vi "Triple coincidence.vi"() -> ()   [LabVIEW 2012]
panel:
  in  "Save file":bool
  in  "Comment":string
  out "Start time":u32
  out "XY Graph":cluster{"Y":dbl[], "Y":dbl[]}[](graph)
  in  "Histogram on/off":bool
  in  "Set window1":bool
  in  "Channel3 Pulse Front":string(combo)
  in  "Channel2 Pulse Front":string(combo)
  out "Waveform Graph 4":cluster{i16, dbl, "Array":i64[]}(graph) caption="Ch1-Ch3"
  out "Waveform Graph 3":cluster{i16, dbl, "Array":i64[]}(graph) caption="Ch1-Ch2"
  out "Waveform Graph 2":cluster{i16, dbl, "Array":i64[]}(graph) caption="Waveform Graph2"
  in  "Window Offset 2 (ns)":i32
  in  "Window Length 2 (ns)":i32
  in  "Window Offset 1 (ns)":i32
  in  "Window Length 1 (ns)":i32
  out "Waveform Graph 1":cluster{i16, dbl, "Array":i64[]}(graph) caption="Waveform Graph"
  out "Single Count Channel3":i64 format="%_3p"
  out "Single Count Channel2":i64 format="%_3p"
  out "Single Count Channel1":i64 format="%_3p"
  out "Exposition time (ms)":i64
  out "Measurement index":i64
  out "Start OK":bool
  in  "Exit":bool
  in  "Channel3 Threshold Voltage (mV)":i32
  in  "Channel2 Threshold Voltage (mV)":i32
  in  "Channel1 Pulse Front":string(combo)
  in  "Channel1 Threshold Voltage (mV)":i32 min=0 max=5000 step=10
  in  "Exposition Time (ms)":i64
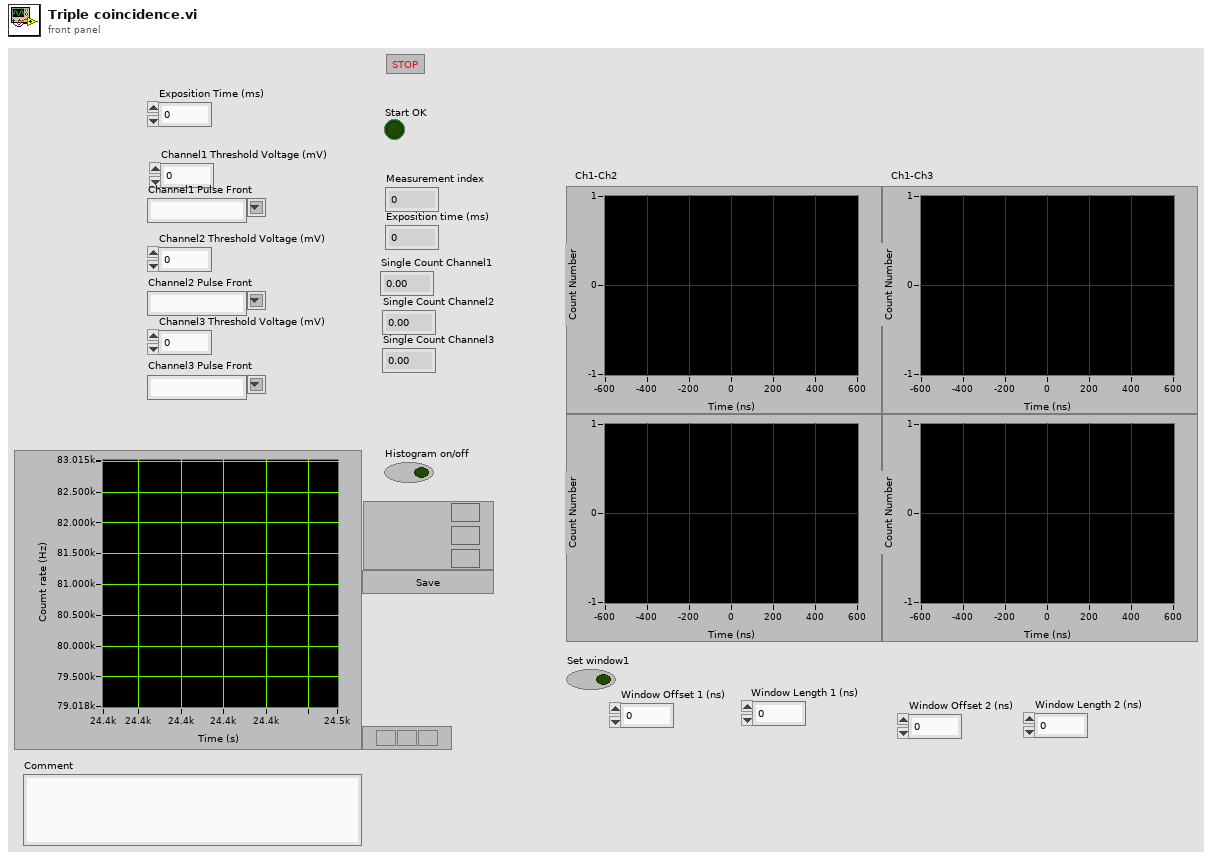
[diagram p1: front panel]
types:
  T1 = cluster{"Channel1":bool, "Channel2":bool, "Channel3":bool, "Channel4":bool}
  T2 = cluster{"Stop Channel":string, "Start Channel":string}
  T3 = cluster{"[0]":i64, "Channel1 Threshold Voltage (mV)":i32, "Channel1 Pulse Front":string, "Channel2 Threshold Voltage (mV)":i32, "Channel2 Pulse Front":string, "Channel3 Threshold Voltage (mV)":i32, "Channel3 Pulse Front ":string, "Channel4 Threshold Voltage (mV)":i32, "Channel4 Pulse Front ":string, "Single Count Enable":cluster{"Channel1":bool, "Channel2":bool, "Channel3":bool, "Channel4":bool}, "Single Count Max":i32, "Sum Count Enable":cluster{"Channel1":bool, "Channel2":bool, "Channel3":bool, "Channel4":bool}, "Sum Count Max":i32, "Start-Stop1 Multyplex":cluster{"Stop Channel":string, "Start Channel":string}, "Stop Delay 1 (ns)":i16, "Window Length 1 (ns)":i32, "Window Offset 1 (ns) ":i32, "Conditional Correlation 1":string, "Histogram Bin 1":string, "Histogram Start 1 (ns) ":i32, "Start-Stop2 Multyplex ":cluster{"Stop Channel":string, "Start Channel":string}, "Stop Delay 2 (ns)":i16, "Window Length 2 (ns) ":i32, "Window Offset 2 (ns) ":i32, "Conditional Correlation 2":string, "Histogram Bin 2":string, "Histogram Start 2 (ns)  ":i32, "Start-Stop3 Multyplex":cluster{"Stop Channel":string, "Start Channel":string}, "Stop Delay 3 (ns)":i16, "Window Length 3 (ns) ":i32, "Window Offset 3 (ns) ":i32, "Conditional Correlation 3":string, "Histogram Bin 3":string, "Histogram Start 3 (ns) ":i32, "Start-Stop4 Multyplex":cluster{"Stop Channel":string, "Start Channel":string}, "Stop Delay 4 (ns)":i16, "Window Length 4 (ns)  ":i32, "Window Offset 4 (ns) ":i32, "Conditional Correlation 4":string, "Histogram Bin 4":string, "Histogram Start 4 (ns)  ":i32, "Coincidence Count Enable":cluster{"Start-Stop1":bool, "Start-Stop2":bool, "Start-Stop3":bool, "Start-Stop4":bool}, "Coincidence Count Max":i32, "Coincidence Sum Enable":cluster{"Start-Stop1":bool, "Start-Stop2":bool, "Start-Stop3":bool, "Start-Stop4":bool}, "Coincidence Sum Max":i32, "Output Channel Enable":cluster{"Channel1":bool, "Channel2":bool, "Channel3":bool, "Channel4":bool}, "Output Channel Inversion":cluster{"Channel1":bool, "Channel2":bool, "Channel3":bool, "Channel4":bool, "Output":bool}}
  T4 = cluster{"Going":bool, "Iinterrupted":bool, "Timer stop":bool, "Single count stop Ch1":bool, "Single count stop Ch2":bool, "Single count stop Ch3":bool, "Single count stop Ch4":bool, "Sum count stop":bool, "Coincidence count stop SS1":bool, "Coincidence count stop SS2":bool, "Coincidence count stop SS3":bool, "Coincidence count stop SS4":bool, "Coincidence sum count stop":bool, "Reserved":bool, "Correlator is not initialised":bool, "Internal error":bool}
  T5 = cluster{"Measurement index":i64, "Exposition time (ms)":i64, "Single Count Channel1":i64, "Single Count Channel2":i64, "Single Count Channel3":i64, "Single Count Channel4":i64, "Sum Single Count":i64, "Coincidence Count SS1":i64, "Coincidence Count SS2":i64, "Coincidence Count SS4":i64, "Coincidence Count SS5":i64, "Sum Coincidence Count":i64}
  T6 = typedef "LVCursorListTypeDef.ctl" = cluster{"Name":string, "Color":u32, "Style":u8, "Point Style":u8, "Name Visible":bool, "Allow Drag":bool, "Cursor Mode":u32, "Plot":i32, "Index":i32, "Position":cluster{"X":dbl, "Y":dbl}, "X Scale":u32, "Y Scale":u32, "Watch Plots":i32[], "Watch All Plots":bool, "Plot Area":i32, "Label Offset":cluster{"X":dbl, "Y":dbl}}[]
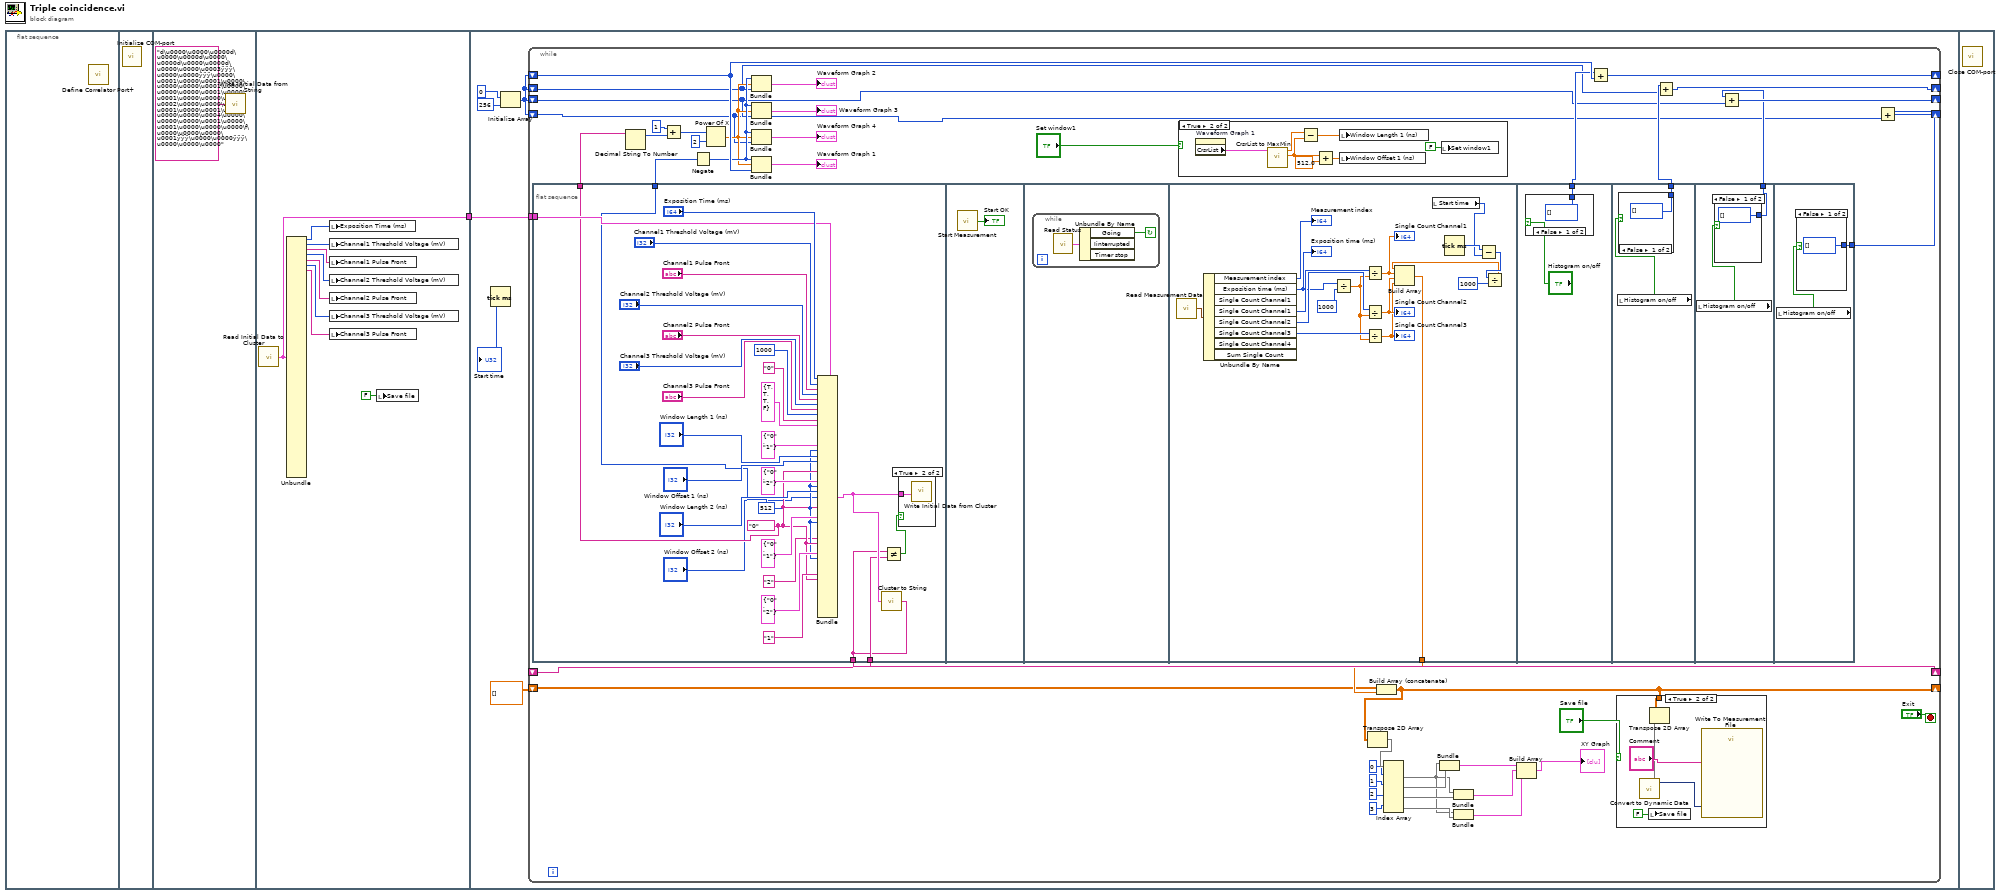
[diagram p0: block diagram]
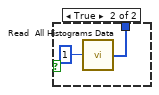
[diagram p5: hidden frame]
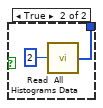
[diagram p6: hidden frame]
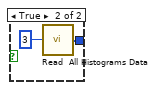
[diagram p7: hidden frame]
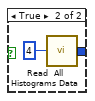
[diagram p8: hidden frame]
diagram:
  n1 = flat-sequence {
    tunnel: [w11] -> w1
    tunnel: w1 -> [w17]
    frame #0 {
      n2 = call "Define Correlator Port+.vi"() -> ()  [unwired: 3 in]
    }
    frame #1 {
      n3 = call "Initialize COM-port.vi"() -> ()  [unwired: 4 in]
    }
    frame #2 {
      n4 = call "Write Initial Data from String.vi"("Data"="d\u0000\u0000\u0000d\u0000\u0000d\u0000\u0000d\u0000\u0000d\u0000\u0000\u0003ÿÿÿ\u0000\u0000ÿÿÿ\u0000\u0001\u0000\u0001\u0000\u0000\u0000\u0001\u0000\u0000\u0000\u0001\u0000\u0001\u0000\u0000\u0000\u0002\u0000\u0000\u0000\u0001\u0000\u0001\u0000\u0000\u0000\u0004\u0000\u0000\u0000\u0001\u0000\u0001\u0000\u0000\u0000\f\u0000\u0000\u0000\u0001ÿÿÿ\u0000\u0000ÿÿÿ\u0000\u0000\u0000") -> ()  [unwired: 1 out]
    }
    frame #3 {
      n5 = call "Read Initial Data to Cluster.vi"() -> ("Correlator Initial Data 2"=w11:T3)  [unwired: 2 in]
      n6 = Unbundle(w11) -> ("[0]"=w10:i64, "Channel1 Threshold Voltage (mV)"=w9:i32, "Channel1 Pulse Front"=w8:string, "Channel2 Threshold Voltage (mV)"=w7:i32, "Channel2 Pulse Front"=w5:string, "Channel3 Threshold Voltage (mV)"=w6:i32, "Channel3 Pulse Front"=w4:string)  [unwired: 40 out]
      n7 = local write "Exposition Time (ms)"(w10) -> ()
      n8 = local write "Channel1 Threshold Voltage (mV)"(w9) -> ()
      n9 = local write "Channel1 Pulse Front"(w8) -> ()
      n10 = local write "Channel2 Threshold Voltage (mV)"(w7) -> ()
      n11 = local write "Channel2 Pulse Front"(w5) -> ()
      n12 = local write "Channel3 Threshold Voltage (mV)"(w6) -> ()
      n13 = local write "Channel3 Pulse Front"(w4) -> ()
      n14 = local write "Save file"(FALSE ("Save file")) -> ()
    }
    frame #4 {
      n15 = Tick Count (ms)() -> (millisecond timer value=→"Start time":u32)
      n16 = Initialize Array(i64 0 ("Value"), 256 ("dimension size")) -> (w14:i64[])
      n17 = while {
        tunnel: w17 -> [w62]
        shift-right: [w61] -> _
        shift-left: w14 -> [w53]
        shift-right: [w46] -> _
        shift-left: w14 -> [w40]
        shift-right: [w45] -> _
        shift-left: w14 -> [w39]
        shift-right: [w41] -> _
        shift-left: w14 -> [w38]
        shift-right: [w37] -> _
        shift-left: _ -> [w36]
        shift-right: [w19] -> _
        shift-left: dbl[][] [] -> [w33]
        stop <- "Exit" stop-if-true
        n18 = flat-sequence {
          tunnel: w62 -> [w97]
          tunnel: [w82] -> w59
          tunnel: [w86] -> w58
          tunnel: [w77] -> w37
          tunnel: w36 -> [w78]
          tunnel: [w112] -> w34
          tunnel: [w125] -> w52
          tunnel: [w130] -> w44
          tunnel: [w135] -> w43
          tunnel: [w140] -> w42
          frame #0 {
            w86 = "0" ("Histogram Bin")
            w82 = i16 512 ("Stop Delay1  (ns)")
            n19 = Bundle(cluster=w97, "[0]"="Exposition Time (ms)", "Channel1 Threshold Voltage (mV)"="Channel1 Threshold Voltage (mV)", "Channel1 Pulse Front"="Channel1 Pulse Front", "Channel2 Threshold Voltage (mV)"="Channel2 Threshold Voltage (mV)", "Channel2 Pulse Front"="Channel2 Pulse Front", "Channel3 Threshold Voltage (mV)"="Channel3 Threshold Voltage (mV)", "Channel3 Pulse Front"="Channel3 Pulse Front", "Channel4 Threshold Voltage (mV)"=1000, "Channel4 Pulse Front"="0", "Single Count Enable"=T1 {"Channel1"=TRUE, "Channel2"=TRUE, "Channel3"=TRUE, "Channel4"=FALSE}, "Start-Stop1 Multyplex"=T2 {"Stop Channel"="0", "Start Channel"="1"}, "Stop Delay 1 (ns)"=w82, "Window Length 1 (ns)"="Window Length 1 (ns)", "Window Offset 1 (ns)"="Window Offset 1 (ns)", "Histogram Bin 1"=w86, "Start-Stop2 Multyplex"=T2 {"Stop Channel"="0", "Start Channel"="2"}, "Stop Delay 2 (ns)"=w82, "Window Length 2 (ns)"="Window Length 2 (ns)", "Window Offset 2 (ns)"="Window Offset 2 (ns)", "Histogram Bin 2"=w86, "Start-Stop3 Multyplex"=T2 {"Stop Channel"="0", "Start Channel"="1"}, "Stop Delay 3 (ns)"=w82, "Conditional Correlation 3"="2", "Histogram Bin 3"=w86, "Start-Stop4 Multyplex"=T2 {"Stop Channel"="0", "Start Channel"="2"}, "Stop Delay 4 (ns)"=w82, "Conditional Correlation 4"="1", "Histogram Bin 4"=w86) -> (w79:T3)  [unwired: 19 in]
            n20 = call "Cluster to String.vi"("Correlator Initial Data"=w79) -> ("string"=w77:string)
            n21 = Not Equal?(x=w77, y=w78) -> (x != y?=w76:bool)
            n22 = case shown="True" w76 {
              tunnel: w79 -> [_ w103]
              frame False {
              }
              frame True {
                n23 = call "Write Initial Data from Cluster.vi"("Correlator Initial Data"=w103) -> ()  [unwired: 2 in, 1 out]
              }
            }
          }
          frame #1 {
            n24 = call "Start Measurement.vi"() -> ("Start OK"=→"Start OK":bool)  [unwired: 2 in]
          }
          frame #2 {
            n25 = while {
              stop <- w105 continue-if-true
              n26 = call "Read Status.vi"() -> ("Status Data"=w106:T4)  [unwired: 2 in]
              n27 = Unbundle By Name(w106) -> ("Going"=w105:bool)  [unwired: 2 out]
            }
          }
          frame #3 {
            n28 = call "Read Measurement Data.vi"() -> ("Measurement Data"=w122:T5)  [unwired: 3 in]
            n29 = Unbundle By Name(w122) -> ("Measurement index"=→"Measurement index":i64, "Exposition time (ms)"=w114:i64, "Single Count Channel1"=w121:i64, "Single Count Channel2"=w118:i64, "Single Count Channel3"=w117:i64)  [unwired: 3 out]
            "Exposition time (ms)" <- w114
            n30 = Divide(x=w114, y=i64 1000) -> (x/y=w115:dbl)
            n31 = Divide(x=w121, y=w115) -> (x/y=w120:dbl)
            "Single Count Channel1" <- w120
            n32 = Divide(x=w118, y=w115) -> (x/y=w119:dbl)
            "Single Count Channel2" <- w119
            n33 = Divide(x=w117, y=w115) -> (x/y=w116:dbl)
            "Single Count Channel3" <- w116
            n34 = local read "Start time"() -> (w110:u32)
            n35 = Tick Count (ms)() -> (millisecond timer value=w111:u32)
            n36 = Subtract(x=w111, y=w110) -> (x-y=w109:u32)
            n37 = Divide(x=w109, y=u32 1000) -> (x/y=w107:dbl)
            n38 = Build Array(w107, w120, w119, w116) -> (w112:dbl[])
          }
          frame #4 {
            n39 = case shown="False" "Histogram on/off" {
              tunnel: [i64[] [] ("Array") w127] -> w125
              frame False {
              }
              frame True {
                n40 = call "Read  All Histograms Data.vi"("Start-Stop#"=i8 1) -> ("Array"=w127:i64[])
              }
            }
          }
          frame #5 {
            n41 = local read "Histogram on/off"() -> (w129:bool)
            n42 = case shown="False" w129 {
              tunnel: [i64[] [] ("Array") w132] -> w130
              frame False {
              }
              frame True {
                n43 = call "Read  All Histograms Data.vi"("Start-Stop#"=i8 2) -> ("Array"=w132:i64[])
              }
            }
          }
          frame #6 {
            n44 = local read "Histogram on/off"() -> (w134:bool)
            n45 = case shown="False" w134 {
              tunnel: [i64[] [] ("Array") w137] -> w135
              frame False {
              }
              frame True {
                n46 = call "Read  All Histograms Data.vi"("Start-Stop#"=i8 3) -> ("Array"=w137:i64[])
              }
            }
          }
          frame #7 {
            n47 = local read "Histogram on/off"() -> (w139:bool)
            n48 = case shown="False" w139 {
              tunnel: [i64[] [] ("Array") w142] -> w140
              frame False {
              }
              frame True {
                n49 = call "Read  All Histograms Data.vi"("Start-Stop#"=i8 4) -> ("Array"=w142:i64[])
              }
            }
          }
        }
        n50 = Decimal String To Number(string=w58) -> (offset past number=w57:i32)  [unwired: 2 in, 1 out]
        n51 = Add(x=1, y=w57) -> (x+y=w54:i32)
        n52 = Negate(x=w59) -> (-x=w48:i16)
        n53 = Power Of X(1:i8 2 ("x"), 2:w54) -> (0:w47:dbl)
        n54 = Bundle(w48, w47, w40) -> (→"Waveform Graph 2":cluster{i16, dbl, i64[]})  [unwired: 1 in]
        n55 = Bundle(w48, w47, w39) -> (→"Waveform Graph 3":cluster{i16, dbl, i64[]})  [unwired: 1 in]
        n56 = Bundle(w48, w47, w38) -> (→"Waveform Graph 4":cluster{i16, dbl, i64[]})  [unwired: 1 in]
        n57 = Bundle(w48, w47, w53) -> (→"Waveform Graph 1":cluster{i16, dbl, i64[]})  [unwired: 1 in]
        n58 = case shown="True" "Set window1" {
          frame False {
          }
          frame True {
            n59 = property on="Waveform Graph 1" class="WFGraph (strict)"() -> ("CrsrList"=w75:T6)  [unwired: 2 in, 2 out]
            n60 = call "CrsrList to MaxMin.vi"("CrsrList"=w75) -> ("Min"=w73:dbl, "Max"=w74:dbl)  [unwired: 9 in]
            n61 = Subtract(x=w74, y=w73) -> (x-y=w71:dbl)
            n62 = Add(x=w73, y=512.0) -> (x+y=w70:dbl)
            n63 = local write "Window Length 1 (ns)"(w71) -> ()
            n64 = local write "Window Offset 1 (ns)"(w70) -> ()
            n65 = local write "Set window1"(FALSE ("Set window1")) -> ()
          }
        }
        n66 = Build Array (concatenate)(w33, w34) -> (w19:dbl[][])
        n67 = Transpose 2D Array(2D array=w19) -> (transposed array=w32:dbl[][])
        n68 = Index Array(array=w32, index (row) #1=0 ("index (row)"), index (row) #2=1 ("disabled index (col)"), index (row) #3=2 ("index (row)"), index (row) #4=3 ("index (row)")) -> (element #1=w24:dbl[], element #2=w27:dbl[], element #3=w26:dbl[], element #4=w25:dbl[])  [unwired: 4 in]
        n69 = Bundle(w24, w27) -> (w23:cluster{dbl[], dbl[]})  [unwired: 1 in]
        n70 = Bundle(w24, w26) -> (w22:cluster{dbl[], dbl[]})  [unwired: 1 in]
        n71 = Bundle(w24, w25) -> (w21:cluster{dbl[], dbl[]})  [unwired: 1 in]
        n72 = Build Array(w23, w22, w21) -> (→"XY Graph":cluster{dbl[], dbl[]}[])
        n73 = Add(x=w52, y=w53) -> (x+y=w61:i64[])
        n74 = case shown="True" "Save file" {
          tunnel: w19 -> [_ w68]
          frame False {
          }
          frame True {
            n75 = local write "Save file"(FALSE ("Save file")) -> ()
            n76 = Transpose 2D Array(2D array=w68) -> (transposed array=w65:dbl[][])
            n77 = call "Convert to Dynamic Data"("2D Array"=w65) -> ("Dynamic Data Type"=w67:dynamicdata)  [unwired: 3 in]
            n78 = call "Write To Measurement File"("Signals"=w67, "Comment"="Comment") -> ()  [unwired: 15 in, 3 out]
          }
        }
        n79 = Add(x=w44, y=w40) -> (x+y=w46:i64[])
        n80 = Add(x=w43, y=w39) -> (x+y=w45:i64[])
        n81 = Add(x=w42, y=w38) -> (x+y=w41:i64[])
      }
    }
    frame #5 {
      n82 = call "Close COM-port.vi"() -> ()  [unwired: 4 in]
    }
  }
